vi "MEASStatus.v.vi"(0 "VisaCluster":T1, 7 "Time (150) ms":u32=150, 11 "error in (no error)":errorcluster) -> (4 "VisaCluster":T1, 8 "Answer":string, 15 "error out":errorcluster)   [LabVIEW 2014, in "FH 55.lvlib"]
doc: "Dieses VI gibt die aktuellen Messwerte des Gaussmeters zurück\n\nThis VI returns the current values of the instrument"
uses:
  FH 55.lvlib
  TypeDef/VisaCluster.ctl
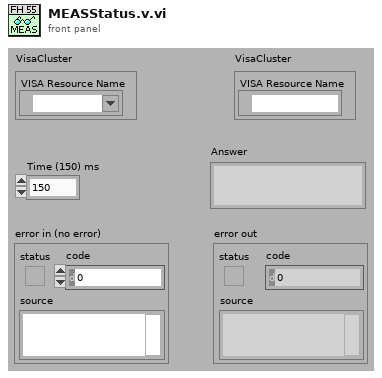
[diagram p1: front panel]
types:
  T1 = typedef "FH 55.lvlib/VisaCluster.ctl" = cluster{"VISA Resource Name":refnum<visa-resource-name>}
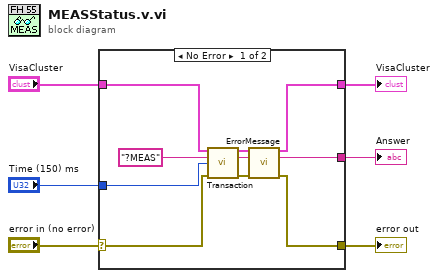
[diagram p0: block diagram]
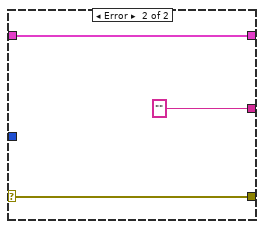
[diagram p2: hidden frame]
diagram:
  n1 = case shown="No Error" "error in (no error)" {
    selector: "error in (no error)" -> [w15 w18]
    tunnel: "VisaCluster" -> [w16 w19]
    tunnel: [w12 w19] -> w2
    tunnel: [w10 w18] -> w4
    tunnel: [w8 ""] -> w3
    tunnel: "Time (150) ms" -> [w7 _]
    frame No Error {
      n2 = call "Transaction.vi"("VisaCluster"=w16, "Command"="?MEAS", "Time (150) ms"=w7, "error in (no error)"=w15) -> ("VisaCluster"=w13:T1, "Answer"=w9:string, "error out"=w11:errorcluster)  [unwired: 8 in, 1 out]
      n3 = call "ErrorMessage.vi"("VisaCluster"=w13, "Message In"=w9, "error in (no error)"=w11) -> ("VisaCluster"=w12:T1, "Message Out"=w8:string, "error out"=w10:errorcluster)  [unwired: 10 in]
    }
    frame Error {
    }
  }
  "error out" <- w4
  "Answer" <- w3
  "VisaCluster" <- w2
